vi "shapeID.vi"(8 "Error":errorcluster, 9 "Nb Circles (Circle Detection 1)":i32, 10 "Circles (Shape Detection 1)":T1(array[cluster]) {"Position"."Y" format="%.2f"; "Position"."X" format="%.2f"}, 11 "KNR in":T2) -> (0 "error out 4":errorcluster caption="error out", 2 "配對數":i32, 3 "KNR out":T2, 5 "配對積木":bool[][](array[boolean]))   [LabVIEW 2013]
uses:
  <userlib>/KNR OS 3.0 LabVIEW Toolkit/Type Definition/KNR3 Reference.ctl
  <userlib>/_FPGA Interface Advanced Tools/FPGA Interface Base/FPGA Interface Base.lvclass
  <userlib>/KNR OS 3.0 LabVIEW Toolkit/Type Definition/Resource.ctl
panel:
  out "sorted array":cluster{"X":sgl, "Y":sgl}[](array[cluster])
  out "影像積木":bool[][](array[boolean])
  out "X中心":sgl
  out "Y中心":sgl
  out "Xmax - Xc":sgl
  out "Xc - Xmin":sgl
  out "Y":sgl
  out "Y 2":sgl
  out "影像積木T.F":bool
  out "配對積木T.F":bool
  out "配對":bool
  out "Ymax - Yc":sgl
  out "L1":sgl
  out "Yc - Ymin":sgl
  out "L2":sgl
  out "0 - 1":sgl
  out "0 - 2":sgl
  out "传1 2":sgl[](array[numeric])
  out "由小到大":sgl[](array[numeric])
  out "x-y 2":sgl
  out "x-y":sgl
  out "Numeric":sgl
  out "Numeric 2":sgl
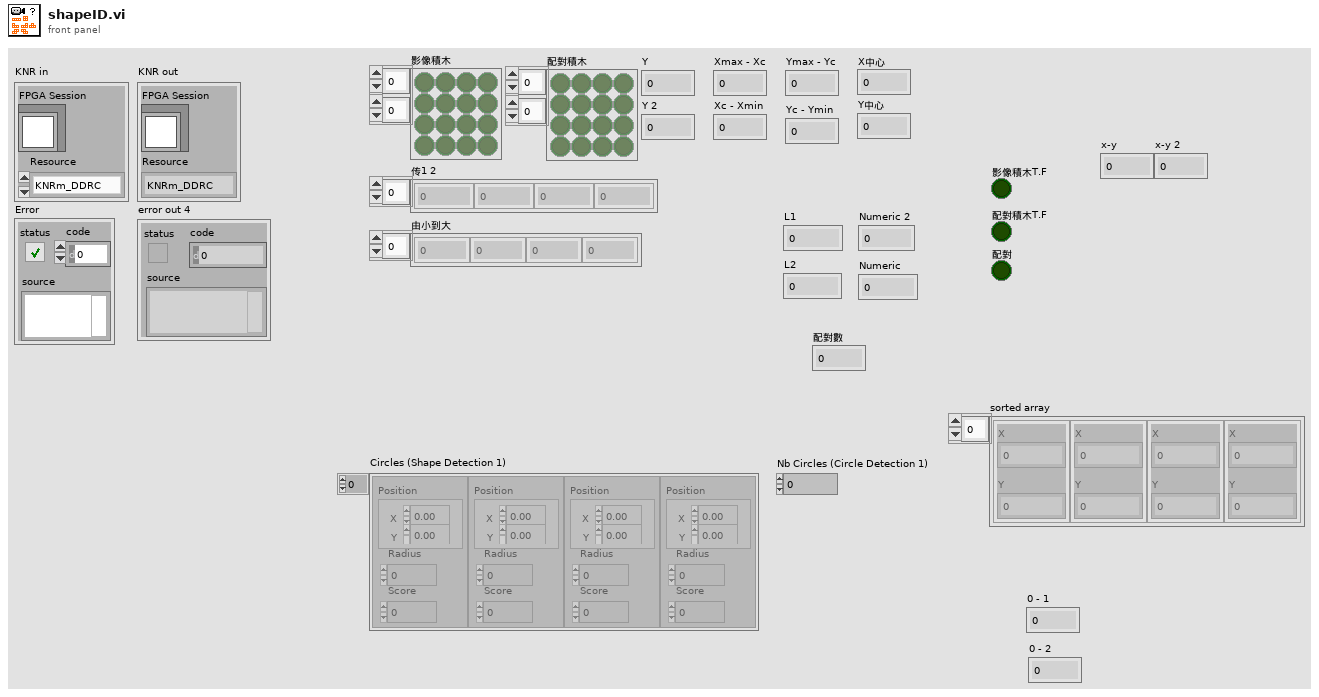
[diagram p1: front panel]
types:
  T1 = cluster{"Position":cluster{"X":sgl, "Y":sgl}, "Radius":dbl, "Score":dbl}[]
  T2 = typedef "KNR3 Reference.ctl" = cluster{"FPGA Session":refnum<class "FPGA Interface Base.lvclass">, "Resource":T3}
  T3 = typedef "Resource.ctl" = enum16{"KNRm_DDRC", "KNRm_DDDD", "KNRm_DDDR", "KNRm_DDDC", "KNR"}
  T4 = cluster{"Position":cluster{"X":sgl, "Y":sgl}, "Radius":dbl, "Score":dbl}
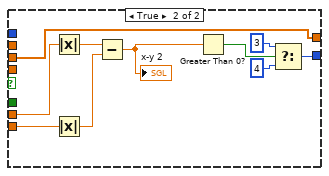
[diagram p3: hidden frame]
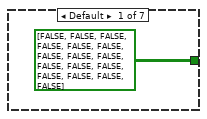
[diagram p4: hidden frame]
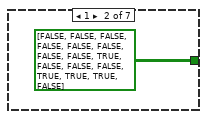
[diagram p5: hidden frame]
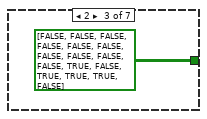
[diagram p6: hidden frame]
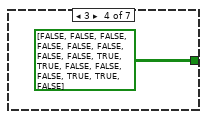
[diagram p7: hidden frame]
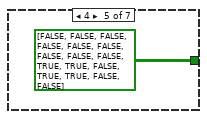
[diagram p8: hidden frame]
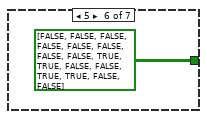
[diagram p9: hidden frame]
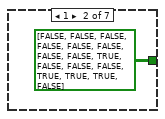
[diagram p10: hidden frame]
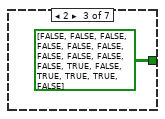
[diagram p11: hidden frame]
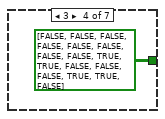
[diagram p12: hidden frame]
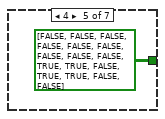
[diagram p13: hidden frame]
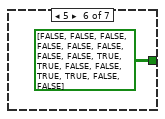
[diagram p14: hidden frame]
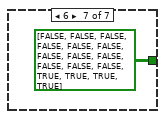
[diagram p15: hidden frame]
diagram:
  n1 = while {
    shift-right: [w146] -> _
    shift-left: 0 -> [w147]
    shift-right: [w148] -> _
    shift-left: 0 -> [w149]
    tunnel: "Circles (Shape Detection 1)" -> [w151]
    tunnel: "Nb Circles (Circle Detection 1)" -> [w150]
    tunnel: "Nb Circles (Circle Detection 1)" -> [w144]
    stop <- w145 stop-if-true
    w114 = 0 ("t")
    n2 = for {
      N: w150 -> [_]
      tunnel: w151 -> [w370]
      tunnel: [w369] -> w67 mode=indexing
      tunnel: [w368] -> w121 mode=indexing
      tunnel: [w367] -> w119 mode=indexing
      i -> [w372]
      n3 = Index Array(array=w370, index=w372) -> (element=w371:T4)
      n4 = Unbundle By Name(w371) -> ("Position.X"=w369:sgl, "Position.Y"=w368:sgl, "Position"=w367:cluster{"X":sgl, "Y":sgl})
    }
    n5 = local read "影像積木"() -> (w105:bool[][])
    n6 = local read "配對積木"() -> (w108:bool[][])
    n7 = local read "配對數"() -> (w142:i32)
    n8 = case shown="Default" w142 {
      tunnel: [bool[][] [[FALSE, FALSE, FALSE, FALSE], [FALSE, FALSE, FALSE, FALSE], [FALSE, FALSE, FALSE, FALSE], [FALSE, FALSE, FALSE, FALSE]] bool[][] [[FALSE, FALSE, FALSE, FALSE], [FALSE, FALSE, FALSE, FALSE], [TRUE, FALSE, FALSE, FALSE], [TRUE, TRUE, TRUE, FALSE]] bool[][] [[FALSE, FALSE, FALSE, FALSE], [FALSE, FALSE, FALSE, FALSE], [FALSE, FALSE, TRUE, FALSE], [TRUE, TRUE, TRUE, FALSE]] bool[][] [[FALSE, FALSE, FALSE, FALSE], [FALSE, FALSE, FALSE, FALSE], [TRUE, TRUE, FALSE, FALSE], [FALSE, TRUE, TRUE, FALSE]] bool[][] [[FALSE, FALSE, FALSE, FALSE], [FALSE, FALSE, FALSE, FALSE], [FALSE, TRUE, TRUE, FALSE], [TRUE, TRUE, FALSE, FALSE]] bool[][] [[FALSE, FALSE, FALSE, FALSE], [FALSE, FALSE, FALSE, FALSE], [TRUE, TRUE, FALSE, FALSE], [TRUE, TRUE, FALSE, FALSE]] bool[][] [[FALSE, FALSE, FALSE, FALSE], [FALSE, FALSE, FALSE, FALSE], [FALSE, FALSE, FALSE, FALSE], [TRUE, TRUE, TRUE, TRUE]]] -> w143
      frame Default {
      }
      frame 1 {
      }
      frame 2 {
      }
      frame 3 {
      }
      frame 4 {
      }
      frame 5 {
      }
      frame 6 {
      }
    }
    "影像積木" <- w143
    n9 = for {
      N: 4 -> [_]
      tunnel: w105 -> [w334]
      shift-right: [w330] -> _
      shift-left: -1 ("disabled index (col)") -> [w326]
      tunnel: w108 -> [w331]
      tunnel: [w327] -> w109
      tunnel: [w324] -> w100
      stop <- w323 stop-if-true
      w328 = -1 ("disabled index (col)")
      n10 = Increment(x=w326) -> (x+1=w325:i32)
      n11 = Greater?(x=w325, y=3) -> (0:w332:bool)
      n12 = Select(t=w325, s=w332, f=w325) -> (s? t:f=w330:i32)
      n13 = for {
        N: 4 -> [_]
        tunnel: w334 -> [w352]
        shift-right: [w350] -> _
        shift-left: w328 -> [w339]
        tunnel: w330 -> [w348]
        shift-right: [w345] -> _
        shift-left: w328 -> [w340]
        tunnel: w331 -> [w344]
        tunnel: w330 -> [w343]
        tunnel: [w335] -> w327
        tunnel: [w335] -> w324
        tunnel: [w335] -> w322
        stop <- w336 stop-if-true
        n14 = Increment(x=w339) -> (x+1=w337:i32)
        n15 = Increment(x=w340) -> (x+1=w338:i32)
        n16 = Greater?(x=w337, y=3) -> (0:w349:bool)
        n17 = Greater?(x=w338, y=3) -> (0:w346:bool)
        n18 = Select(t=w337, s=w349, f=w337) -> (s? t:f=w350:i32)
        n19 = Select(t=w338, s=w346, f=w338) -> (s? t:f=w345:i32)
        n20 = Index Array(array=w352, index (row)=w348, index (col)=w350) -> (element=w342:bool)
        "影像積木T.F" <- w342
        n21 = Index Array(array=w344, index (row)=w343, index (col)=w345) -> (element=w341:bool)
        "配對積木T.F" <- w341
        n22 = Equal?(x=w342, y=w341) -> (x = y?=w335:bool)
        "配對" <- w335
        n23 = Not(x=w335) -> (.not. x?=w336:bool)
      }
      n24 = Not(x=w322) -> (.not. x?=w323:bool)
    }
    n25 = Sort 1D Array(array=w119) -> (sorted array=w118:cluster{"X":sgl, "Y":sgl}[])
    "sorted array" <- w118
    n26 = Index Array(array=w67, index #1=0 ("index"), index #2=1 ("index"), index #3=2 ("index"), index #4=3 ("index")) -> (element #1=w141:sgl, element #2=w140:sgl, element #3=w139:sgl, element #4=w138:sgl)
    n27 = Index Array(array=w121, index #1=0 ("index"), index #2=1 ("index"), index #3=2 ("index"), index #4=3 ("index")) -> (element #1=w122:sgl, element #2=w123:sgl, element #3=w124:sgl, element #4=w125:sgl)
    n28 = Index Array(array=w118, index #1=0 ("index"), index #2=1 ("index"), index #3=2 ("index"), index #4=3 ("index")) -> (element #1=w115:cluster{"X":sgl, "Y":sgl}, element #2=w8:cluster{"X":sgl, "Y":sgl}, element #3=w7:cluster{"X":sgl, "Y":sgl}, element #4=w9:cluster{"X":sgl, "Y":sgl})
    n29 = Compound Arithmetic op=ADD(w141, w140, w139, w138) -> (w133:sgl)
    n30 = Compound Arithmetic op=ADD(w122, w123, w124, w125) -> (w130:sgl)
    n31 = Unbundle By Name(w115) -> ("Y"=w64:sgl)
    "Y 2" <- w64
    n32 = Unbundle By Name(w8) -> ("X"=w89:sgl, "Y"=w65:sgl)
    n33 = Unbundle By Name(w7) -> ("X"=w87:sgl, "Y"=w66:sgl)
    n34 = Unbundle By Name(w9) -> ("Y"=w63:sgl)
    "Y" <- w63
    n35 = Divide(x=w133, y=sgl 4.0) -> (x/y=w120:sgl)
    "X中心" <- w120
    n36 = Divide(x=w130, y=sgl 4.0) -> (x/y=w69:sgl)
    "Y中心" <- w69
    n37 = Array Max & Min(array=w67) -> (max value=w88:sgl, min value=w62:sgl)  [unwired: 2 out]
    n38 = Subtract(x=w88, y=w120) -> (x-y=w74:sgl)
    "Xmax - Xc" <- w74
    n39 = Subtract(x=w120, y=w62) -> (x-y=w73:sgl)
    "Xc - Xmin" <- w73
    n40 = Subtract(x=w69, y=w64) -> (x-y=w95:sgl)
    "Yc - Ymin" <- w95
    n41 = Subtract(x=w62, y=w89) -> (x-y=w86:sgl)
    n42 = Subtract(x=w62, y=w87) -> (x-y=w85:sgl)
    n43 = Subtract(x=w64, y=w65) -> (x-y=w84:sgl)
    n44 = Subtract(x=w63, y=w69) -> (x-y=w99:sgl)
    "Ymax - Yc" <- w99
    n45 = Subtract(x=w64, y=w66) -> (x-y=w83:sgl)
    n46 = Square(x=w86) -> (x^2=w82:sgl)
    n47 = Square(x=w84) -> (x^2=w81:sgl)
    n48 = Square(x=w85) -> (x^2=w80:sgl)
    n49 = Square(x=w83) -> (x^2=w79:sgl)
    n50 = Add(x=w82, y=w81) -> (x+y=w78:sgl)
    n51 = Add(x=w80, y=w79) -> (x+y=w77:sgl)
    n52 = Square(x=w74) -> (x^2=w98:sgl)
    n53 = Square(x=w73) -> (x^2=w94:sgl)
    n54 = Square(x=w95) -> (x^2=w93:sgl)
    n55 = Square(x=w99) -> (x^2=w97:sgl)
    n56 = Add(x=w98, y=w97) -> (x+y=w96:sgl)
    n57 = Add(x=w94, y=w93) -> (x+y=w92:sgl)
    n58 = Square Root(x=w78) -> (sqrt(x)=w76:sgl)
    "0 - 1" <- w76
    n59 = Square Root(x=w77) -> (sqrt(x)=w75:sgl)
    "0 - 2" <- w75
    n60 = Square Root(x=w96) -> (sqrt(x)=w72:sgl)
    "L1" <- w72
    n61 = Square Root(x=w92) -> (sqrt(x)=w71:sgl)
    "L2" <- w71
    n62 = Sort 1D Array(array=w67) -> (sorted array=w68:sgl[])
    n63 = flat-sequence {
      tunnel: w149 -> [w176]
      tunnel: w74 -> [w164]
      tunnel: w73 -> [w163]
      tunnel: [w178] -> w61
      tunnel: [w166] -> w60
      tunnel: [w165] -> w59
      tunnel: w72 -> [w166]
      tunnel: w71 -> [w165]
      tunnel: [w164] -> w58
      tunnel: [w163] -> w57
      tunnel: w76 -> [w162]
      tunnel: [w162] -> w56
      tunnel: w75 -> [w154]
      tunnel: [w154] -> w55
      tunnel: w69 -> [w161]
      tunnel: [w161] -> w54
      tunnel: w65 -> [w155]
      tunnel: [w155] -> w53
      tunnel: w68 -> [w160]
      tunnel: [w160] -> w52
      tunnel: [w159] -> w51
      tunnel: w69 -> [w159]
      tunnel: w72 -> [w157]
      tunnel: [w157] -> w50
      tunnel: w71 -> [w156]
      tunnel: [w156] -> w49
      tunnel: [w152] -> w48
      tunnel: w66 -> [w152]
      tunnel: w65 -> [w153]
      tunnel: [w153] -> w47
      tunnel: w61 -> [w204]
      tunnel: [w194] -> w46
      tunnel: w60 -> [w193]
      tunnel: w59 -> [w192]
      tunnel: [w193] -> w45
      tunnel: [w192] -> w44
      tunnel: w58 -> [w191]
      tunnel: w57 -> [w190]
      tunnel: w56 -> [w189]
      tunnel: [w189] -> w43
      tunnel: w55 -> [w188]
      tunnel: [w188] -> w42
      tunnel: [w187] -> w41
      tunnel: w54 -> [w187]
      tunnel: [w186] -> w40
      tunnel: w53 -> [w186]
      tunnel: [w185] -> w39
      tunnel: w52 -> [w185]
      tunnel: w51 -> [w184]
      tunnel: [w184] -> w38
      tunnel: w50 -> [w182]
      tunnel: [w182] -> w37
      tunnel: w49 -> [w181]
      tunnel: [w181] -> w36
      tunnel: [w180] -> w35
      tunnel: w48 -> [w180]
      tunnel: w47 -> [w179]
      tunnel: [w179] -> w34
      tunnel: w46 -> [w228]
      tunnel: w45 -> [w218]
      tunnel: w44 -> [w217]
      tunnel: [w219] -> w33
      tunnel: [w218] -> w32
      tunnel: [w217] -> w31
      tunnel: [w216] -> w30
      tunnel: w43 -> [w216]
      tunnel: w42 -> [w215]
      tunnel: [w215] -> w29
      tunnel: [w214] -> w28
      tunnel: w41 -> [w214]
      tunnel: [w211] -> w27
      tunnel: w40 -> [w211]
      tunnel: [w213] -> w26
      tunnel: w39 -> [w213]
      tunnel: [w212] -> w25
      tunnel: w38 -> [w212]
      tunnel: [w209] -> w24
      tunnel: w37 -> [w209]
      tunnel: [w208] -> w23
      tunnel: w36 -> [w208]
      tunnel: w35 -> [w206]
      tunnel: [w206] -> w22
      tunnel: w34 -> [w207]
      tunnel: [w207] -> w21
      tunnel: w33 -> [w252]
      tunnel: w32 -> [w247]
      tunnel: w31 -> [w242]
      tunnel: [w241] -> w20
      tunnel: w30 -> [w241]
      tunnel: w29 -> [w231]
      tunnel: [w231] -> w19
      tunnel: [w240] -> w18
      tunnel: w28 -> [w240]
      tunnel: [w239] -> w17
      tunnel: w27 -> [w239]
      tunnel: w26 -> [w238]
      tunnel: [w238] -> w16
      tunnel: [w237] -> w15
      tunnel: w25 -> [w237]
      tunnel: [w236] -> w14
      tunnel: [w235] -> w13
      tunnel: w24 -> [w235]
      tunnel: [w234] -> w12
      tunnel: w23 -> [w234]
      tunnel: w22 -> [w233]
      tunnel: [w233] -> w11
      tunnel: w21 -> [w232]
      tunnel: [w232] -> w10
      tunnel: [w257] -> w148
      tunnel: w20 -> [w256]
      tunnel: w19 -> [w255]
      tunnel: w18 -> [w280]
      tunnel: w17 -> [w279]
      tunnel: w16 -> [w278]
      tunnel: w15 -> [w275]
      tunnel: w14 -> [w273]
      tunnel: w13 -> [w264]
      tunnel: w12 -> [w263]
      tunnel: w11 -> [w259]
      tunnel: w10 -> [w258]
      frame #0 {
        # "L"
        n64 = Less?(x=w164, y=w163) -> (x < y?=w167:bool)
        n65 = Greater Or Equal?(x=w166, y=30.0 ("x")) -> (x >= y?=w174:bool)
        n66 = Less?(x=w166, y=60.0 ("x")) -> (x < y?=w171:bool)
        n67 = Greater Or Equal?(x=w165, y=50.0 ("x")) -> (x >= y?=w172:bool)
        n68 = Less?(x=w165, y=68.0 ("x")) -> (x < y?=w170:bool)
        n69 = Compound Arithmetic op=AND(w174, w171, w172, w170, w167) -> (w158:bool)
        n70 = Select(t=i16 2 ("y"), s=w158, f=w176) -> (s? t:f=w178:i32)
      }
      frame #1 {
        # "J"
        n71 = Greater?(x=w191, y=w190) -> (0:w203:bool)
        n72 = Greater Or Equal?(x=w193, y=45.0 ("x")) -> (x >= y?=w195:bool)
        n73 = Less?(x=w193, y=66.0 ("x")) -> (x < y?=w196:bool)
        n74 = Greater Or Equal?(x=w192, y=28.0 ("x")) -> (x >= y?=w199:bool)
        n75 = Less?(x=w192, y=45.0 ("x")) -> (x < y?=w200:bool)
        n76 = Compound Arithmetic op=AND(w195, w196, w199, w200, w203) -> (w183:bool)
        n77 = Select(t=i16 1 ("y"), s=w183, f=w204) -> (s? t:f=w194:i32)
      }
      frame #2 {
        # "I"
        n78 = Greater Or Equal?(x=w218, y=60.0 ("x")) -> (x >= y?=w220:bool)
        n79 = Less?(x=w218, y=76.0) -> (x < y?=w222:bool)
        n80 = Greater Or Equal?(x=w217, y=60.0 ("x")) -> (x >= y?=w225:bool)
        n81 = Less?(x=w217, y=76.0) -> (x < y?=w226:bool)
        n82 = Compound Arithmetic op=AND(w220, w222, w225, w226) -> (w210:bool)
        n83 = Select(t=i16 6 ("y"), s=w210, f=w228) -> (s? t:f=w219:i32)
      }
      frame #3 {
        # "O"
        n84 = Greater Or Equal?(x=w247, y=sgl 30.0) -> (x >= y?=w251:bool)
        n85 = Less?(x=w247, y=sgl 40.0) -> (x < y?=w249:bool)
        n86 = Greater Or Equal?(x=w242, y=sgl 30.0) -> (x >= y?=w246:bool)
        n87 = Less?(x=w242, y=sgl 40.0) -> (x < y?=w243:bool)
        n88 = Compound Arithmetic op=AND(w251, w249, w246, w243) -> (w230:bool)
        n89 = Select(t=i16 5 ("y"), s=w230, f=w252) -> (s? t:f=w236:i32)
      }
      frame #4 {
        # "Z"
        # "S"
        n90 = Greater?(x=w255, y=w256) -> (0:w254:bool)
        n91 = Greater?(x=w279, y=w280) -> (0:w277:bool)
        n92 = Greater Or Equal?(x=w264, y=sgl 50.0) -> (x >= y?=w268:bool)
        n93 = Less?(x=w264, y=60.0) -> (x < y?=w269:bool)
        n94 = Greater Or Equal?(x=w263, y=sgl 50.0) -> (x >= y?=w270:bool)
        n95 = Less?(x=w263, y=60.0) -> (x < y?=w271:bool)
        n96 = Compound Arithmetic op=AND(w268, w269, w270, w271) -> (w262:bool)
        n97 = Compound Arithmetic op=AND(w268, w269, w270, w271) -> (w261:bool)
        n98 = Or(x=w262, y=w261) -> (x .or. y?=w260:bool)
        n99 = case shown="True" w260 {
          tunnel: w278 -> [w281 w292]
          tunnel: w277 -> [_ w291]
          tunnel: [w282 w290] -> w257
          tunnel: [w281 w289] -> w276
          tunnel: w275 -> [_ w288]
          tunnel: dbl[] [0.0, 0.0, 0.0, 0.0] -> [_ w287]
          tunnel: w254 -> [_ w286]
          tunnel: w273 -> [w282 w285]
          tunnel: w259 -> [_ w284]
          tunnel: w258 -> [_ w283]
          frame False {
          }
          frame True {
            n100 = case shown="False" w286 {
              tunnel: w292 -> [w310 w318]
              tunnel: w285 -> [_ _]
              tunnel: w291 -> [_ _]
              tunnel: [w297 w321] -> w290
              tunnel: [w300 w318] -> w289
              tunnel: w288 -> [_ _]
              tunnel: w287 -> [w305 _]
              tunnel: w284 -> [w294 w315]
              tunnel: w283 -> [w293 w312]
              frame False {
                n101 = Subtract(x=w294, y=w293) -> (x-y=w296:sgl)
                "x-y" <- w296
                n102 = Index Array(array=w310, index #1=0, index #2=1, index #3=2, index #4=3) -> (element #1=w304:sgl, element #2=w303:sgl, element #3=w302:sgl, element #4=w301:sgl)
                n103 = Greater Than 0?(x=w296) -> (x > 0?=w295:bool)
                n104 = Insert Into Array(array=w305, index=0, new element #1=w304, new element #2=w302, new element #3=w303, new element #4=w301) -> (w300:dbl[])
                n105 = Select(t=4 ("index"), s=w295, f=3) -> (s? t:f=w297:i32)
              }
              frame True {
                n106 = Absolute Value(x=w315) -> (abs(x)=w314:sgl)
                n107 = Absolute Value(x=w312) -> (abs(x)=w313:sgl)
                n108 = Subtract(x=w314, y=w313) -> (x-y=w317:sgl)
                "x-y 2" <- w317
                n109 = Greater Than 0?(x=w317) -> (x > 0?=w316:bool)
                n110 = Select(t=3, s=w316, f=4) -> (s? t:f=w321:i32)
              }
            }
          }
        }
        "配對數" <- w257
        "传1 2" <- w276
        "由小到大" <- w278
        "Numeric" <- w255
        "Numeric 2" <- w256
      }
    }
    n111 = Increment(x=w147) -> (x+1=w110:i32)
    n112 = Less?(x=w144, y=4 ("t")) -> (x < y?=w104:bool)
    n113 = Greater?(x=w144, y=4 ("t")) -> (0:w103:bool)
    n114 = case shown="6" w110 {
      tunnel: [bool[][] [[FALSE, FALSE, FALSE, FALSE], [FALSE, FALSE, FALSE, FALSE], [FALSE, FALSE, FALSE, FALSE], [FALSE, FALSE, FALSE, FALSE]] bool[][] [[FALSE, FALSE, FALSE, FALSE], [FALSE, FALSE, FALSE, FALSE], [TRUE, FALSE, FALSE, FALSE], [TRUE, TRUE, TRUE, FALSE]] bool[][] [[FALSE, FALSE, FALSE, FALSE], [FALSE, FALSE, FALSE, FALSE], [FALSE, FALSE, TRUE, FALSE], [TRUE, TRUE, TRUE, FALSE]] bool[][] [[FALSE, FALSE, FALSE, FALSE], [FALSE, FALSE, FALSE, FALSE], [TRUE, TRUE, FALSE, FALSE], [FALSE, TRUE, TRUE, FALSE]] bool[][] [[FALSE, FALSE, FALSE, FALSE], [FALSE, FALSE, FALSE, FALSE], [FALSE, TRUE, TRUE, FALSE], [TRUE, TRUE, FALSE, FALSE]] bool[][] [[FALSE, FALSE, FALSE, FALSE], [FALSE, FALSE, FALSE, FALSE], [TRUE, TRUE, FALSE, FALSE], [TRUE, TRUE, FALSE, FALSE]] bool[][] [[FALSE, FALSE, FALSE, FALSE], [FALSE, FALSE, FALSE, FALSE], [FALSE, FALSE, FALSE, FALSE], [TRUE, TRUE, TRUE, TRUE]]] -> w70
      frame Default {
      }
      frame 1 {
      }
      frame 2 {
      }
      frame 3 {
      }
      frame 4 {
      }
      frame 5 {
      }
      frame 6 {
      }
    }
    "配對積木" <- w70
    n115 = Select(t=w114, s=w109, f=w110) -> (s? t:f=w113:i32)
    n116 = Compound Arithmetic op=OR(w104, w103, w100) -> (w145:bool)
    n117 = Greater Or Equal?(x=w110, y=6) -> (x >= y?=w112:bool)
    n118 = Select(t=w114, s=w112, f=w113) -> (s? t:f=w146:i32)
  }
  "KNR out" <- "KNR in"
  "error out 4" <- "Error"
